vi "AppConfigTypeToXML.vi"(8 "error in (no error)":errorcluster, 11 "LSEPlugin in":refnum<class "LSEPlugin.lvclass">) -> (0 "error out":errorcluster, 2 "ConfigXML out":string, 3 "LSEPlugin out":refnum<class "LSEPlugin.lvclass">)   [LabVIEW 2014, in "AppPlugins.lvlib" / "LSEPlugin.lvclass"]
uses:
  LSEPlugin.lvclass
  PublicAPI/Typedefs/LSEConfig.ctl
  LSEPlugin.lvclass/LSEPlugin.ctl
  Accessors/Read LSEConfig.vi
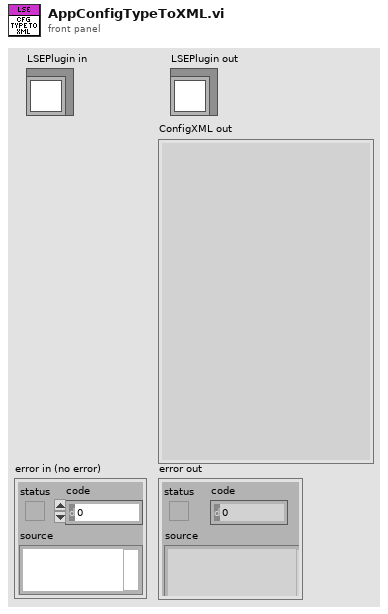
[diagram p1: front panel]
types:
  T1 = typedef "AppPlugins.lvlib/LSEPlugin.lvclass/LSEConfig.ctl" = cluster{"NoiseVariance":dbl, "IEEESystem":u32, "PMULocations":u32[], "Vindex":i32, "Iindex":i32, "DynamicRef":string}
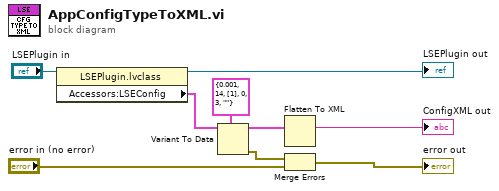
[diagram p0: block diagram]
diagram:
  n1 = property class="LSEPlugin.lvclass"(reference="LSEPlugin in") -> (reference out=→"LSEPlugin out":refnum<class "LSEPlugin.lvclass">, "Accessors:LSEConfig"=w5:T1)  [unwired: 1 in, 1 out]
  n2 = Variant To Data(type=T1 {"NoiseVariance"=0.001, "IEEESystem"=14, "PMULocations"=[1], "Vindex"=0, "Iindex"=3, "DynamicRef"=""} ("LSEConfig"), Variant=w5) -> (data=w3:T1, error out=w1:errorcluster)  [unwired: 1 in]
  n3 = Flatten To XML(anything=w3) -> (xml string=→"ConfigXML out":string)
  n4 = Merge Errors(w1, "error in (no error)") -> (→"error out":errorcluster)
